vi "Time.Secs to H_M_S Duration.vi"(10 "Total Secs":dbl format="%#.3f") -> (2 "Duration(HH:MM:SS)":string)   [LabVIEW 2019]
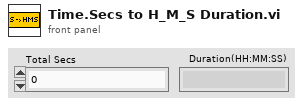
[diagram p1: front panel]
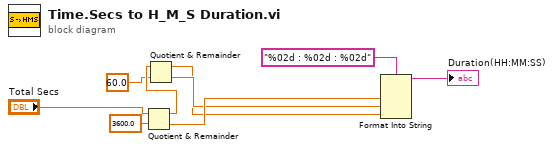
[diagram p0: block diagram]
diagram:
  n1 = Quotient & Remainder(x="Total Secs", y=3600.0) -> (x-y*floor(x/y)=w8:dbl, floor(x/y)=w4:dbl)
  n2 = Quotient & Remainder(x=w8, y=60.0) -> (x-y*floor(x/y)=w2:dbl, floor(x/y)=w3:dbl)
  n3 = Format Into String(format string="%02d : %02d : %02d", w4, w3, w2) -> (resulting string=→"Duration(HH:MM:SS)":string)  [unwired: 2 in, 1 out]
